vi "plot_spectrum.vi"(0 "reference":refnum<class "OSA.lvclass">, 4 "autoScale Y":bool, 5 "error in (no error)":errorcluster, 7 "skip":bool, 9 "error rangeViolation":bool) -> (14 "duplicate reference":refnum<class "OSA.lvclass">, 19 "error out":errorcluster={"status"=TRUE, "code"=5000, "source"="\nNot enough nr of data points in acqusition or plot data.\r\n[Thorlabs_FTS_LV61_plot_data_update.vi->Thorlabs_FTS_LV61_plot_update.vi->Thorlabs_FTS_LV61_plot_spectrum.vi->Thorlabs_FTS_LV61_example_asyncAcqusition.vi]"})   [LabVIEW 2010, in "OSA.lvclass"]
doc: "This will write a plot in an intensity graph if a corresponding reference has been provided/routed to init.vi. A compatible graph to copy can be found in the tree.vi."
uses:
  OSA.lvclass
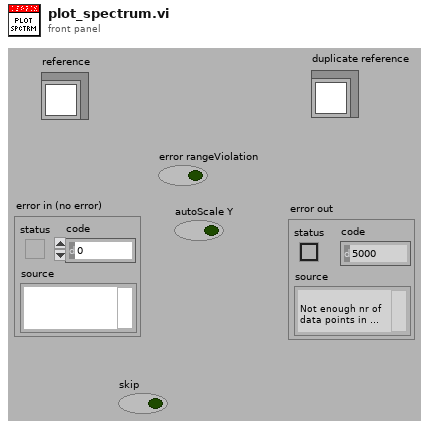
[diagram p1: front panel]
types:
  T1 = enum16{"get", "init", "set interferogram", "set spectrum", "cleanUp"}
  T2 = typedef "OSA.lvclass/ObjectAttributes.ctl" = cluster{"Stop":bool, "dataType":T3, "spectrometerIdx":u16, "buffer size interferogram":i32, "interferogram":cluster{"new":bool, "plot_x_ min":sgl, "plot_x_max":sgl, "plot_y_min":sgl, "plot_y_max":sgl, "Graph Intrfrgrm":T4, "timeStamp":u32, "signal (%)":dbl, "traces":cluster{"idx":u32, "broadBand":bool, "monoChromatic":bool, "peakToPeakSignal":dbl, "peakToPeakPos":dbl}[], "traces idx last":i32, "contrast (%)":dbl}, "spectrum":cluster{"new":bool, "plot_x_min":sgl, "plot_x_max":sgl, "plot_unit_x":T5, "plot_unit_y":T6, "plot_y_min":sgl, "plot_y_max":sgl, "Graph Spectrum":T4, "timeStamp":u32, "X_VAL_OPTIONS":enum16{"MIN_MAX", "ARRAY"}, "traces":cluster{"idx":u32}[], "traces idx last":i32}, "Thorlabs_OSA_64.lvclass:queue_action.ctlqueue ref":refnum<queue>, "action":T7, "plot zoom step":dbl, "buffer semaphore":T8, "acq stopped":bool, "dataType active":T3, "temperature (degr C)":sgl, "pressure (hPa)":sgl, "rel humidity (%)":sgl, "settings":cluster{"resolution":u16, "sensitivity":u16, "Average":bool, "average nr":u32, "apodisation":T9, "acq delay (ms)":u32, "airMesure":T10, "wmtr on":bool, "intfgrm_smooth_width":u16, "intfgrm_smooth_nrOfPasses":u16, "intfgrm_smooth":T11, "phaseCorrection":T12, "zeroFill":u8, "spectr_smooth":T11, "spectr_smooth_width":u16, "spectr_smooth_nrOfPasses":u16, "resolution (/cm)":sgl, "REF wavelength, (nm)":dbl, "gain_idx":u16, "gainAuto":bool, "gain_relative":dbl, "PD sensitivity mode":T13, "PD senseMode implemented":bool, "SensorTemperature implemented":bool, "SensorPressure implemented":bool, "SensorHumidity implemented":bool, "attenuationAuto":bool, "attenuationOnOff":bool, "attenuationAvailable":bool, "offsetAvailable":bool, "offset":i32, "offset max":u16, "contrastAvailable":bool}, "peaks position":sgl[], "peaks width":sgl[], "peaks height":sgl[], "peaks max nr":u32, "peaks latest nr":i32, "peaks new":bool, "power":dbl, "power new":bool, "path":string, "wavelength (WNr)":dbl, "wavelength new":bool, "buffer size spectrum":i32, "status":string, "vi reference":refnum<vi>, "funcPointer":u64, "libraryPointer":u64, "singleAcquisition":bool, "coherenceLength (cm)":dbl, "coherenceLength new":bool, "spectrometer model":string, "spectrometer serial nr":string, "peaks thld left":sgl[], "peaks thld right":sgl[], "coherenceLength error (cm)":dbl, "ADC bits":u16, "peaks position centroid":sgl[], "peaks height centroid":sgl[], "OSA series":T14, "channel index spectrum":u16, "spectrometer rangeLow, (/cm)":dbl, "spectrometer rangeHigh, (/cm)":dbl, "channel index interferogram":u16, "virtualSource":bool, "sweep restart":bool}
  T3 = typedef "OSA.lvclass/acq_dataType.ctl" = enum16{"none", "interferogram", "spectrum"}
  T4 = typedef "OSA.lvclass/graph_intensity.ctl" = refnum<vi>
  T5 = typedef "OSA.lvclass/spectrum_x_unit.ctl" = enum16{"wavenr/cm", "THz", "eV", "nm_air", "nm_vac"}
  T6 = typedef "OSA.lvclass/y_unit.ctl" = enum16{"ADC counts", "dBm pwr absolute", "dBm pwr density", "mW pwr absolute", "mW pwr density"}
  T7 = typedef "OSA.lvclass/queue_action.ctl" = enum16{"none", "stop", "GUI_plotInterferogram", "GUI_plotSpectrum", "GUI_plotInterferogramRescale", "GUI_plotSpectrumRescale", "GUI_plotInterferogramReset", "GUI_plotSpectrumReset", "GUI_plotInterferogramAutoScaleY", "GUI_plotSpectrumAutoScaleY", "GUI_plotInterferogramZoomOut", "GUI_plotSpectrumZoomOut", "GUI_plotInterferogramPane", "GUI_plotSpectrumPane", "GUI_plotInterferogramZoomMouse", "GUI_plotSpectrumZoomMouse", "GUI_plotSpectrumFSRY", "GUI_plotInterferogramFSRY", "GUI_spectrumChannelType", "GUI_channel", "ENVIRONMENT temperature", "ENVIRONMENT pressure", "MODE_resolution set", "MODE_resolution get", "MODE_sensitivity set", "MODE_sensitivity get", "MODE_PDTemperature set", "MODE_PDTemperature get", "REBOOT/RESET firmware", "ACQASYNC_acquireSingleSpectrum", "ACQASYNC_continuous start", "ACQASYNC_continuous stop\n", "ACQASYNC_get last interferogram", "ACQASYNC_get last spectrum", "ACQASYNC_get last waveNr", "ACQOPT_interferogram smoothing set", "ACQOPT_interferogram smoothing get", "ACQOPT_spectrum smoothing set", "ACQOPT_spectrum smoothing get", "ACQOPT_apodisation type set", "ACQOPT_apodisation type get", "ACQOPT_phase correction type set", "ACQOPT_phase correction type get", "ACQOPT_acqIntervall_set", "ACQOPT_acqIntervall_get", "ACQOPT_average spectrum set", "ACQOPT_average spectrum get", "ACQOPT_rolling average set", "ACQOPT_rolling average get", "ACQOPT_zero fill factor set", "ACQOPT_zero fill factor get", "ACQOPT_cycle counting set", "ACQOPT_cycle counting get", "ACQOPT_air measure option set", "ACQOPT_air measure option get", "ACQOPT_gainLevel auto get", "ACQOPT_gainLevel auto set", "ACQOPT_gainLevel get", "ACQOPT_gainLevel set", "ACQOPT_offset set", "ACQOPT_attenuator_auto_set", "ACQOPT_attenuator_set", "ACQOPT_getAll", "INSTRUMENT_PROPERTY_range_WaveNr_min", "INSTRUMENT_PROPERTY_range_WaveNr_max", "INSTRUMENT_PROPERTY_reference_wavelength_cm^-1", "INSTRUMENT_PROPERTY_samplesPerRefPeriod", "INSTRUMENT_PROPERTY_resolution_waveNrPercm", "INSTRUMENT_PROPERTY_availableGainLevels", "INSTRUMENT_PROPERTY_status", "CONVERT", "ANALYSE_POWER", "ANALYSE_PEAKS", "ANALYSE_WAVELENGTH", "ANALYSE_SPECTRUM", "ANALYSE_INTERFEROGRAM", "ANALYSE_COHERENCE_LENGTH", "MATH", "MATH_power", "MATH_peaks", "FILE", "miscellaneous"}
  T8 = typedef "Semaphore RefNum" = refnum<k1>
  T9 = typedef "OSA.lvclass/apodisation.ctl" = enum16{"NONE", "NORTON_BEER_WEAK", "NORTON_BEER_MEDIUM", "NORTON_BEER_STRONG", "TRIANGULAR", "COSINE", "HANN", "HAMMING", "BLACKMANHARRIS3", "BLACKMANHARRIS4", "GAUSSIAN"}
  T10 = typedef "OSA.lvclass/airMeasure.ctl" = enum16{"TEMPERATURE", "PRESSURE"}
  T11 = typedef "OSA20X_misc.lvlib/interferogram_smoothing.ctl" = enum16{"NONE", "BINOMIAL", "SAVITSKY_GOLAY", "FOURIER", "MOVING_AVERAGE", "GAUSSIAN"}
  T12 = typedef "OSA.lvclass/phaseCorrection.ctl" = enum16{"NONE", "MERTZ", "FORMAN", "MERTZ_FILE", "FORMAN_FILE", "FUTURE COMP."}
  T13 = typedef "OSA20X_misc.lvlib/PDTemperatureMode.ctl" = enum16{"cool: better sensitivity/noise floor", "warm: extended wl range"}
  T14 = typedef "OSA.lvclass/OSA_series.ctl" = enum16{"OSA200", "OSA300", "UNKNOWN"}
  T15 = cluster{"new":bool, "plot_x_min":sgl, "plot_x_max":sgl, "plot_unit_x":T5, "plot_unit_y":T6, "plot_y_min":sgl, "plot_y_max":sgl, "Graph Spectrum":T4, "timeStamp":u32, "X_VAL_OPTIONS":enum16{"MIN_MAX", "ARRAY"}, "traces":cluster{"idx":u32}[], "traces idx last":i32}
  T16 = typedef "OSA.lvclass/spectrum_properties.ctl" = cluster{"length":u32, "X min":sgl, "X max":sgl, "X_VAL_OPTIONS":T17}
  T17 = typedef "OSA.lvclass/xVal_option.ctl" = enum16{"MIN_MAX", "ARRAY"}
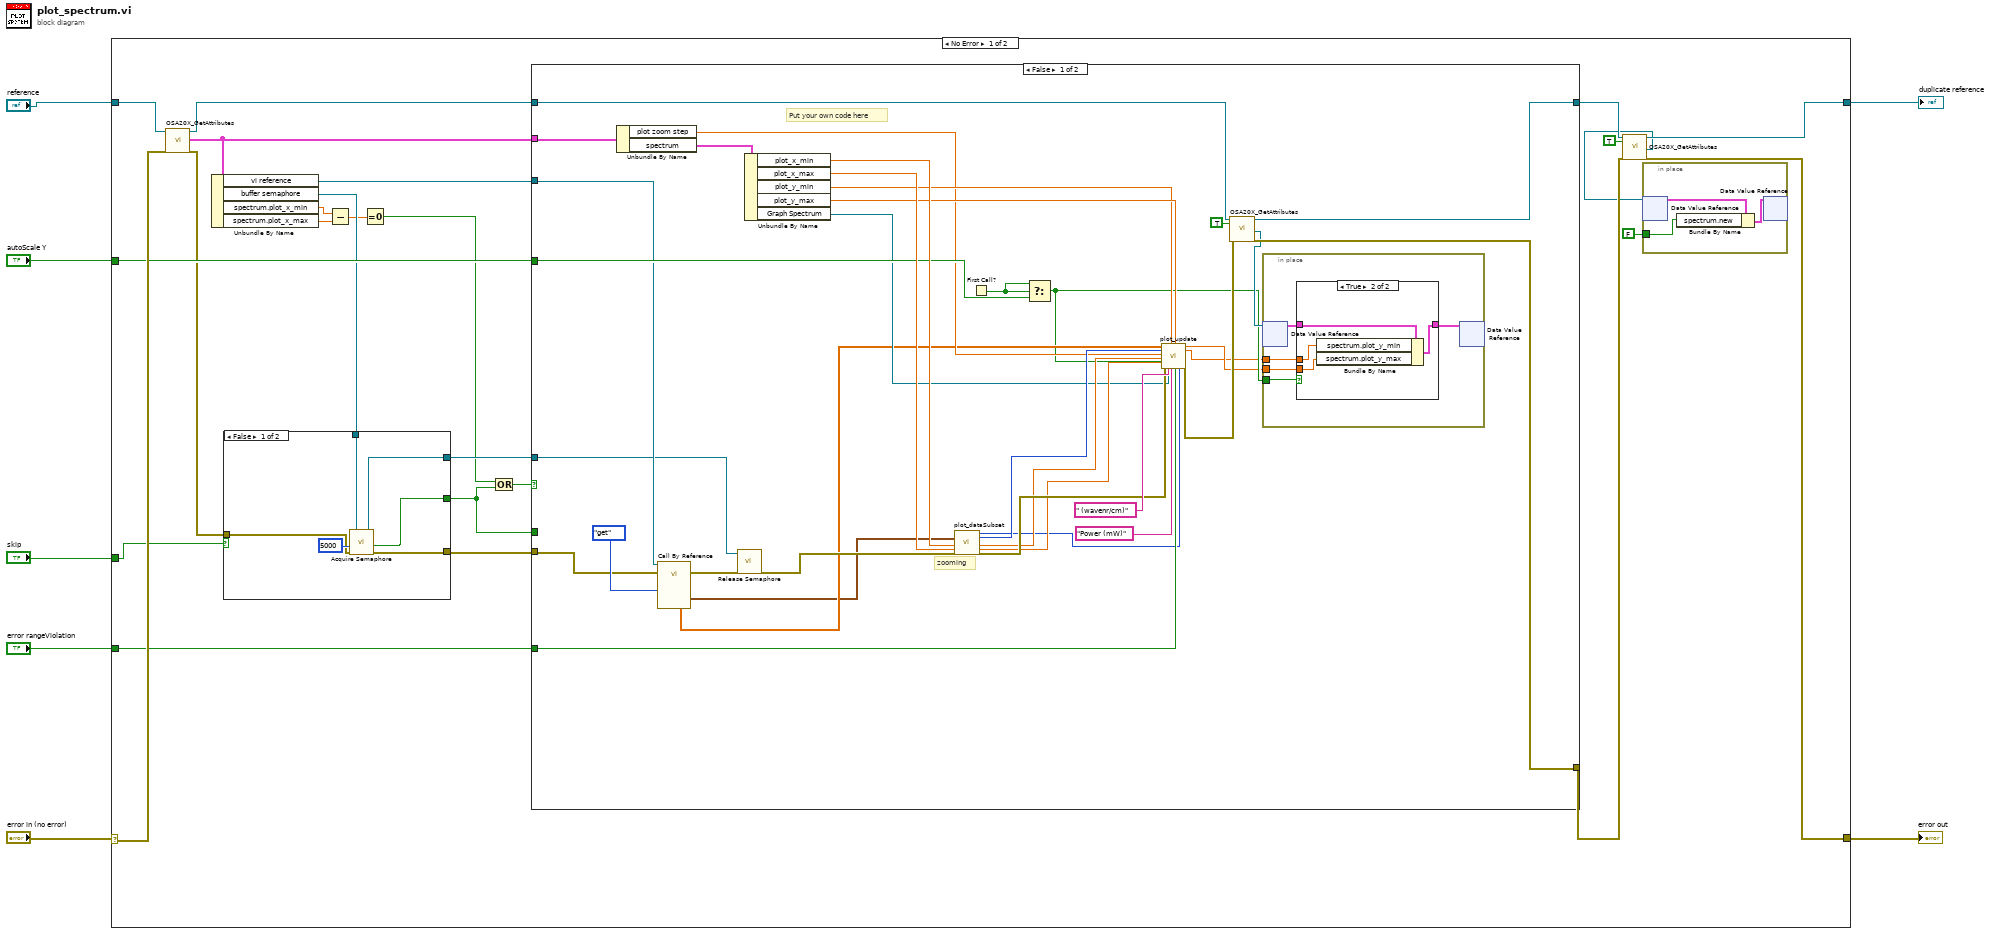
[diagram p0: block diagram]
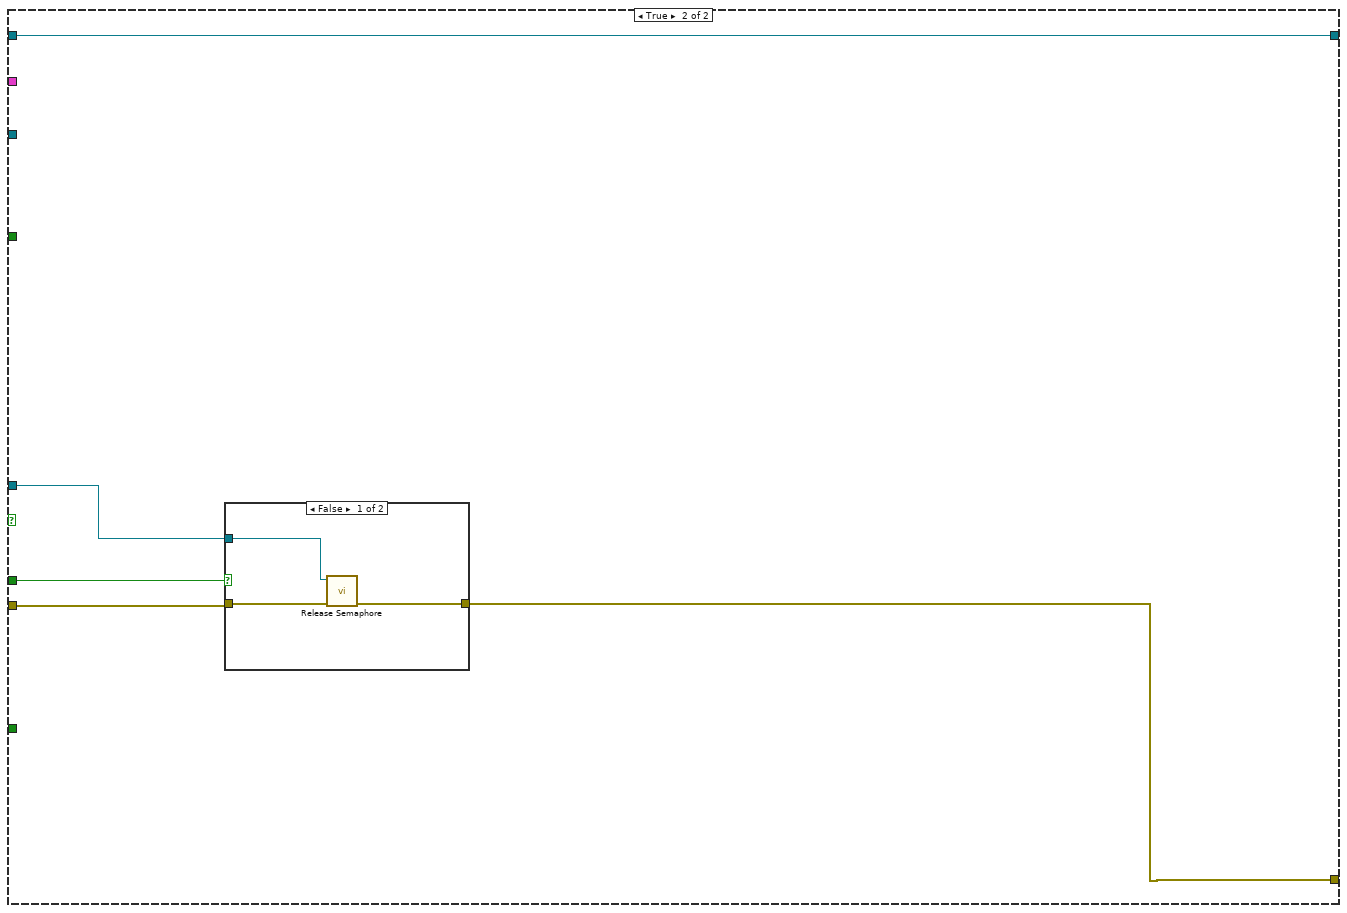
[diagram p4: hidden frame]
diagram:
  n1 = case shown="No Error" "error in (no error)" {
    selector: "error in (no error)" -> [w31 w99]
    tunnel: [w27 w99] -> w7
    tunnel: "reference" -> [w32 w100]
    tunnel: [w26 w100] -> w4
    tunnel: "error rangeViolation" -> [w30 _]
    tunnel: "autoScale Y" -> [w29 _]
    tunnel: "skip" -> [w24 _]
    frame No Error {
      n2 = call "OSA20X_GetAttributes.vi"("reference in"=w32, "error in (no error)"=w31) -> ("reference out"=w20:refnum<class "OSA.lvclass">, "Data"=w10:T2, "error out"=w22:errorcluster)  [unwired: 14 in, 1 out]
      n3 = Unbundle By Name(w10) -> ("vi reference"=w18:refnum<vi>, "buffer semaphore"=w19:T8, "spectrum.plot_x_min"=w15:sgl, "spectrum.plot_x_max"=w14:sgl)
      n4 = case shown="False" w24 {
        selector: w24 -> [_ w44]
        tunnel: w19 -> [w41 w43]
        tunnel: [w36 w44] -> w12
        tunnel: [w39 w43] -> w23
        tunnel: w22 -> [w38 w42]
        tunnel: [w37 w42] -> w21
        frame False {
          n5 = call <vilib>:"Acquire Semaphore.vi"("error in (no error)"=w38, "ms timeout (-1)"=5000, "semaphore"=w41) -> ("error out"=w37:errorcluster, "timed out"=w36:bool, "semaphore out"=w39:T8)  [unwired: 2 in]
        }
        frame True {
        }
      }
      n6 = Subtract(x=w15, y=w14) -> (x-y=w16:sgl)
      n7 = Equal To 0?(x=w16) -> (x = 0?=w13:bool)
      n8 = Or(x=w13, y=w12) -> (x .or. y?=w17:bool)
      n9 = case shown="False" w17 {
        tunnel: [w77 w94] -> w25
        tunnel: [w75 w90] -> w28
        tunnel: w10 -> [w74 _]
        tunnel: w30 -> [w66 _]
        tunnel: w29 -> [w62 _]
        tunnel: w23 -> [w54 w92]
        tunnel: w21 -> [w56 w91]
        tunnel: w18 -> [w55 _]
        tunnel: w20 -> [w53 w94]
        tunnel: w12 -> [_ w93]
        frame False {
          # "zooming"
          # "Put your own code here"
          n10 = Unbundle By Name(w74) -> ("plot zoom step"=w61:dbl, "spectrum"=w73:T15)
          n11 = call-by-ref "?"(reference=w55, error in=w56, "action"=T1."get") -> (error out=w58:errorcluster, "spectrum Y"=w52:sgl[], "spectrum prop"=w45:T16)  [unwired: 14 in, 4 out]
          n12 = call <vilib>:"Release Semaphore.vi"("error in (no error)"=w58, "semaphore"=w54) -> ("error out"=w57:errorcluster)  [unwired: 4 in, 1 out]
          n13 = Unbundle By Name(w73) -> ("plot_x_min"=w71:sgl, "plot_x_max"=w70:sgl, "plot_y_min"=w64:sgl, "plot_y_max"=w65:sgl, "Graph Spectrum"=w60:T4)
          n14 = call "plot_dataSubset.vi"("spectrum property"=w45, "zoom range low"=w71, "zoom range high"=w70, "error in (no error)"=w57) -> ("idx start"=w51:i32, "length"=w69:i32, "X min actual"=w68:sgl, "X max actual"=w67:sgl, "error out"=w72:errorcluster)  [unwired: 11 in]
          n15 = First Call?() -> (First Call?: T/F=w63:bool)
          n16 = Select(t=w63, s=w63, f=w62) -> (s? t:f=w48:bool)
          n17 = call "plot_update.vi"("data"=w52, "data length"=w69, "x zoom factor"=w61, "X range min"=w68, "X range max"=w67, "error in (no error)"=w72, "graph ref"=w60, "X Scale.Name Label.Text"=" (wavenr/cm)", "y min value"=w64, "Y Scale.Name Label.Text"="Power (mW)", "y max value"=w65, "error rangeViolation"=w66, "autoScale Y"=w48, "data idxStart"=w51) -> ("dataVal max"=w47:sgl, "dataVal min"=w46:sgl, "error out"=w76:errorcluster)  [unwired: 3 in]
          n18 = call "OSA20X_GetAttributes.vi"("reference in"=w53, "OnlyGetDvrReference(False)"=TRUE, "error in (no error)"=w76) -> ("reference out"=w77:refnum<class "OSA.lvclass">, "DataRef"=w49:refnum<data-value>, "error out"=w75:errorcluster)  [unwired: 13 in, 1 out]
          n19 = in-place {
            in-place-border: w48 -> [w84]
            in-place-border: w47 -> [w82]
            in-place-border: w46 -> [w81]
            n20 = in-place-dvr #1(w49) -> (w83:T2)  [unwired: 1 out]
            n21 = case shown="True" w84 {
              tunnel: w83 -> [w85 w89]
              tunnel: [w85 w88] -> w80
              tunnel: w82 -> [_ w87]
              tunnel: w81 -> [_ w86]
              frame False {
              }
              frame True {
                n22 = Bundle By Name(cluster=w89, "spectrum.plot_y_min"=w86, "spectrum.plot_y_max"=w87) -> (w88:T2)
              }
            }
            n23 = in-place-dvr #1(w80) -> ()  [unwired: 2 out]
          }
        }
        frame True {
          n24 = case shown="False" w93 {
            tunnel: w92 -> [w97 _]
            tunnel: w91 -> [w96 w98]
            tunnel: [w95 w98] -> w90
            frame False {
              n25 = call <vilib>:"Release Semaphore.vi"("error in (no error)"=w96, "semaphore"=w97) -> ("error out"=w95:errorcluster)  [unwired: 4 in, 1 out]
            }
            frame True {
            }
          }
        }
      }
      n26 = call "OSA20X_GetAttributes.vi"("reference in"=w25, "OnlyGetDvrReference(False)"=TRUE, "error in (no error)"=w28) -> ("reference out"=w26:refnum<class "OSA.lvclass">, "DataRef"=w9:refnum<data-value>, "error out"=w27:errorcluster)  [unwired: 13 in, 1 out]
      n27 = in-place {
        in-place-border: FALSE ("dataNewIntrfrgrm") -> [w34]
        n28 = in-place-dvr #2(w9) -> (w35:T2)  [unwired: 1 out]
        n29 = Bundle By Name(cluster=w35, "spectrum.new"=w34) -> (w33:T2)
        n30 = in-place-dvr #2(w33) -> ()  [unwired: 2 out]
      }
    }
    frame Error {
      # "Error"
    }
  }
  "error out" <- w7
  "duplicate reference" <- w4
